vi "calc centroid and save to tdms.vi"(8 "error in (no error)":errorcluster, 9 "Range":cluster{"Lower value":sgl, "Upper value":sgl}, 10 "Image Out":T1, 11 "Refnum in":refnum<k34>) -> (0 "error out":errorcluster, 3 "Refnum out":refnum<k34>)   [LabVIEW 2020]
uses:
  <vilib>/vision/NI_Vision_Development_Module.lvlib
  <vilib>/vision/Image Controls.llb/IMAQ Image.ctl
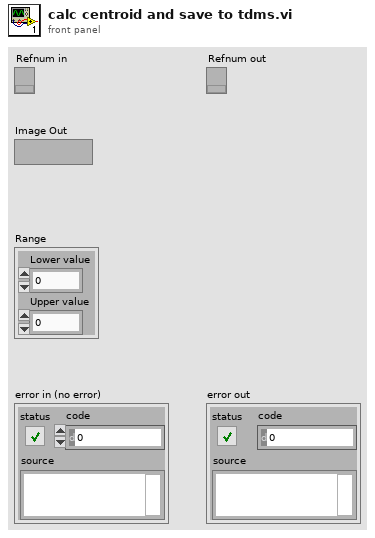
[diagram p1: front panel]
types:
  T1 = typedef "IMAQ Image.ctl" = refnum<image>
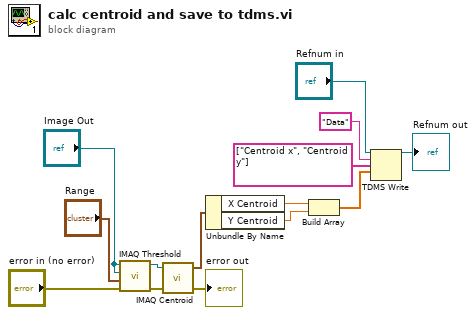
[diagram p0: block diagram]
diagram:
  n1 = call "IMAQ Threshold"("error in (no error)"="error in (no error)", "Range"="Range", "Image Dst"="Image Out", "Image Src"="Image Out") -> ("error out"=w6:errorcluster, "Image Dst Out"=w5:T1)  [unwired: 6 in]
  n2 = call "IMAQ Centroid"("error in (no error)"=w6, "Image"=w5) -> ("error out"=→"error out":errorcluster, "Centroid"=w12:cluster{"X Centroid":sgl, "Y Centroid":sgl})  [unwired: 2 in]
  n3 = Unbundle By Name(w12) -> ("X Centroid"=w13:sgl, "Y Centroid"=w2:sgl)
  n4 = Build Array(w13, w2) -> (w1:sgl[])
  n5 = TDMS Write(0:"Refnum in", 5:"Data" ("group name in (Untitled)"), 7:string[] ["Centroid x", "Centroid y"] ("channel name(s) in (Untitled)"), 9:w1) -> (4:→"Refnum out":refnum<k34>)  [unwired: 2 in, 3 out]
